vi "HEWH Totalize Flow Control.vi"(0 "VISA session":refnum<visa-resource-name>="MW100", 7 "Totalize Flow":bool, 11 "error in (no error)":errorcluster) -> (4 "dup VISA session":refnum<visa-resource-name>="MW100", 15 "error out":errorcluster)   [LabVIEW 2016]
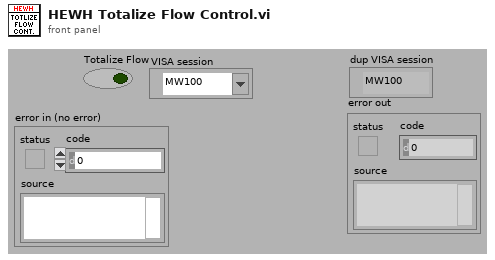
[diagram p1: front panel]
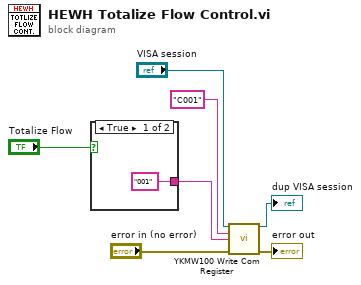
[diagram p0: block diagram]
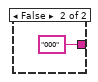
[diagram p2: hidden frame]
diagram:
  n1 = case shown="True" "Totalize Flow" {
    tunnel: ["001" ("Channel") "000" ("Channel")] -> w6
    frame True {
    }
    frame False {
    }
  }
  n2 = call "YKMW100 Write Com Register.vi"("VISA session"="VISA session", "Channel"="C001", "Value"=w6, "error in (no error)"="error in (no error)") -> ("dup VISA session"=→"dup VISA session":refnum<visa-resource-name>, "error out"=→"error out":errorcluster)  [unwired: 10 in]
